vi "uTransport_uActor_Destroy.vi"(8 "error in (no error)":errorcluster, 11 "uTransport_uActor in":refnum<class "uTransport_uActor.lvclass">) -> (0 "error out":errorcluster, 2 "remaining elements":refnum<class "uMsg.lvclass">[](array[class]))   [LabVIEW 2021, in "uFramework.lvlib" / "uTransport_uActor.lvclass"]
uses:
  uTransport_uActor.lvclass
  uMsg/uMsg.lvclass
  uTransport_uActor.lvclass/uTransport_uActor.ctl
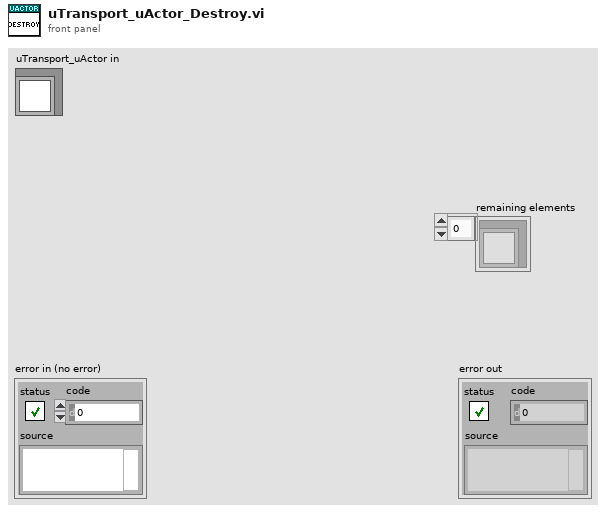
[diagram p1: front panel]
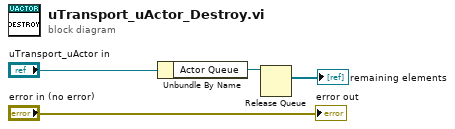
[diagram p0: block diagram]
diagram:
  n1 = Unbundle By Name("uTransport_uActor in") -> ("Actor Queue"=w4:refnum<queue>)
  n2 = Release Queue(queue=w4) -> (remaining elements=→"remaining elements":refnum<class "uMsg.lvclass">[])  [unwired: 2 in, 2 out]
  "error out" <- "error in (no error)"
